vi "Write File to Parse.vi"(8 "error in (no error)":errorcluster, 10 "File to Parse":path, 11 "File Parsing Interface in":refnum<class "File Parsing Interface.lvclass">) -> (0 "error out":errorcluster, 3 "File Parsing Interface out":refnum<class "File Parsing Interface.lvclass">)   [LabVIEW 2018, in "File Parsing Interface.lvlib" / "File Parsing Interface.lvclass"]
uses:
  File Parsing Interface.lvclass
  File Parsing Interface.lvclass/File Parsing Interface.ctl
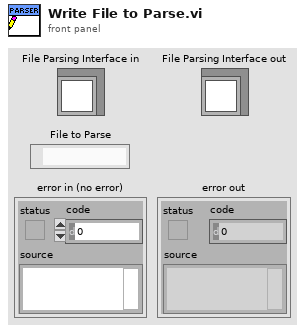
[diagram p1: front panel]
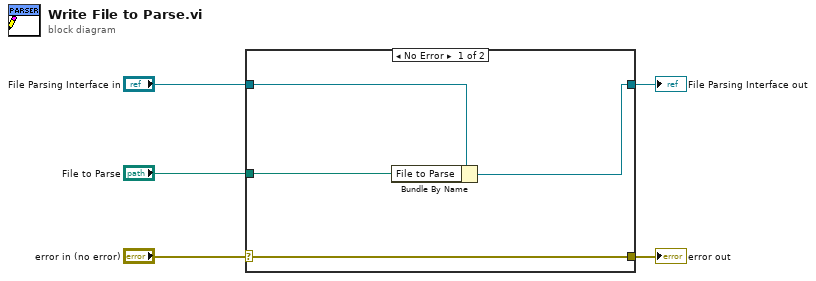
[diagram p0: block diagram]
diagram:
  n1 = case shown="No Error" "error in (no error)" {
    selector: "error in (no error)" -> [w6 w10]
    tunnel: [w6 w10] -> w4
    tunnel: [w7 w11] -> w2
    tunnel: "File Parsing Interface in" -> [w9 w11]
    tunnel: "File to Parse" -> [w8 _]
    frame No Error {
      n2 = Bundle By Name(cluster=w9, "File to Parse"=w8) -> (w7:refnum<class "File Parsing Interface.lvclass">)
    }
    frame Error {
    }
  }
  "error out" <- w4
  "File Parsing Interface out" <- w2
